vi "data_logger_temp.vi"() -> ()   [LabVIEW 2020]
panel:
  in  "VISA resource name":refnum<visa-resource-name>
  in  "Data Records":string[][](table)
  out "Humidity":dbl(graph)
  out "Temperature":dbl(graph)
  out "Humidity":dbl(knob) scale=0.0..100.0
  out "Temp":dbl(slide) scale=0.0..100.0
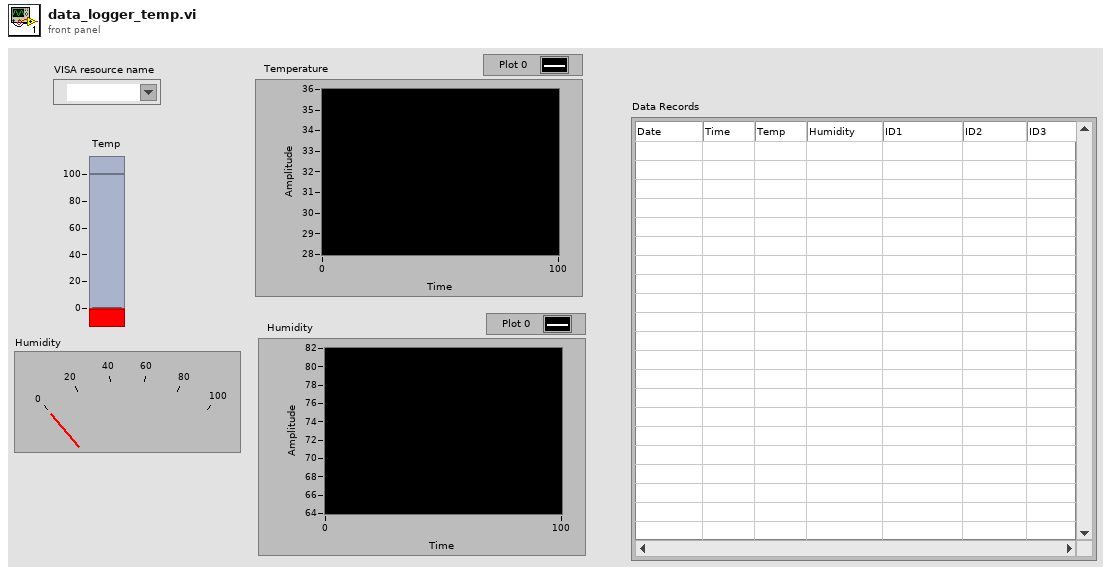
[diagram p1: front panel]
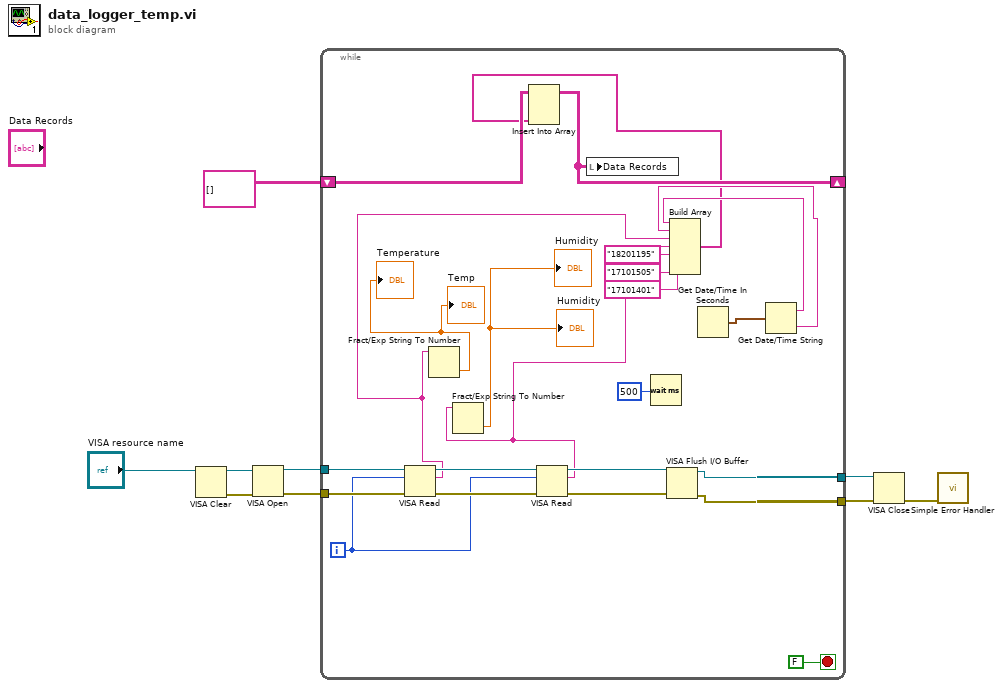
[diagram p0: block diagram]
diagram:
  n1 = VISA Clear(VISA resource name="VISA resource name") -> (VISA resource name out=w4:refnum<visa-resource-name>, error out=w3:errorcluster)  [unwired: 1 in]
  n2 = VISA Open(error in (no error)=w3, VISA resource name=w4) -> (VISA resource name=w9:refnum<visa-resource-name>, error out=w8:errorcluster)  [unwired: 3 in]
  n3 = while {
    tunnel: w9 -> [w33]
    tunnel: w8 -> [w32]
    tunnel: [w27] -> w7
    tunnel: [w26] -> w6
    shift-right: [w22] -> _
    shift-left: string[][] [] -> [w23]
    i -> [w25]
    stop <- FALSE stop-if-true
    n4 = VISA Read(VISA resource name=w33, byte count=w25, error in (no error)=w32) -> (VISA resource name out=w31:refnum<visa-resource-name>, read buffer=w16:string, error out=w30:errorcluster)  [unwired: 1 out]
    n5 = Fract/Exp String To Number(string=w16) -> (number=→"Temp" →"Temperature":dbl)  [unwired: 3 in, 1 out]
    n6 = VISA Read(VISA resource name=w31, byte count=w25, error in (no error)=w30) -> (VISA resource name out=w29:refnum<visa-resource-name>, read buffer=w15:string, error out=w28:errorcluster)  [unwired: 1 out]
    n7 = Fract/Exp String To Number(string=w15) -> (number=→"Humidity" →"Humidity":dbl)  [unwired: 3 in, 1 out]
    n8 = Wait (ms)(milliseconds to wait=u32 500 ("millisecond timer value")) -> ()  [unwired: 1 out]
    n9 = VISA Flush I/O Buffer(VISA resource name=w29, error in (no error)=w28) -> (VISA resource name out=w27:refnum<visa-resource-name>, error out=w26:errorcluster)  [unwired: 1 in]
    n10 = Get Date/Time In Seconds() -> (seconds since 1Jan1904=w19:timestamp)
    n11 = Get Date/Time String(seconds (now)=w19) -> (date string=w18:string, time string=w17:string)  [unwired: 2 in]
    n12 = Build Array(w18, w17, w16, w15, "18201195" ("element"), "17101505" ("element"), "17101401" ("element")) -> (w10:string[])
    n13 = Insert Into Array(array=w23, new element=w10) -> (w22:string[][])  [unwired: 2 in]
    n14 = local write "Data Records"(w22) -> ()
  }
  n15 = VISA Close(VISA resource name=w7, error in (no error)=w6) -> (error out=w5:errorcluster)
  n16 = call <vilib>:"Simple Error Handler.vi"("error in (no error)"=w5) -> ()  [unwired: 4 in, 5 out]
